vi "P4CMD Find All Providers.vi"(8 "error in (no error)":errorcluster) -> (0 "error out":errorcluster, 1 "additional data":string[](array[string]), 2 "provider locations":string[](array[string]), 3 "provider names":string[](array[string]))   [LabVIEW 2020, in "NI_SCC_P4CMD.lvlib"]
uses:
  <vilib>/SourceControl/Providers/P4CMD/NI_SCC_P4CMD.lvlib
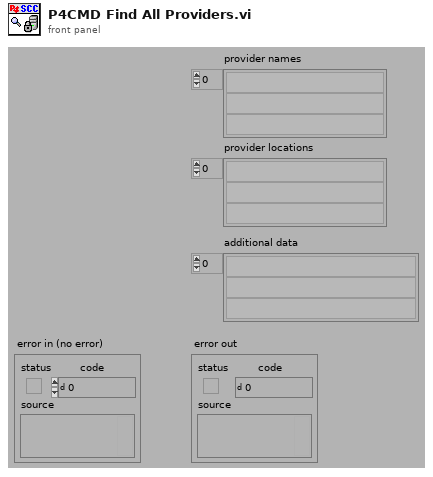
[diagram p1: front panel]
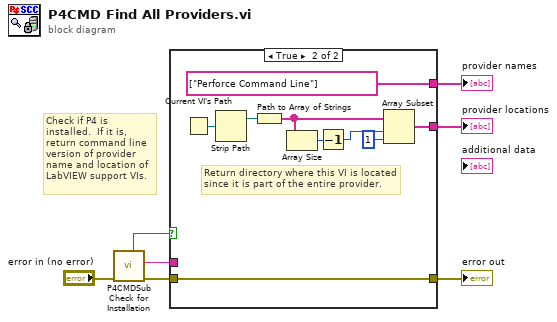
[diagram p0: block diagram]
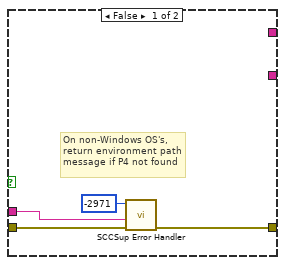
[diagram p2: hidden frame]
diagram:
  # "Check if P4 is installed.  If it is, return command line version of provider name and location of LabVIEW support VIs."
  n1 = call <vilib>:"P4CMDSub Check for Installation.vi"("error in (no error)"="error in (no error)") -> ("error out"=w2:errorcluster, "path info"=w4:string, "Perforce installed?"=w5:bool)  [unwired: 8 in]
  n2 = case shown="True" w5 {
    tunnel: [_ string[] ["Perforce Command Line"] ("provider names")] -> w7
    tunnel: w4 -> [w9 _]
    tunnel: [_ w12] -> w3
    tunnel: w2 -> [w11 w19]
    tunnel: [w10 w19] -> w1
    frame False {
      # "On non-Windows OS's, return environment path message if P4 not found"
      n3 = call <vilib>:"SCCSup Error Handler.vi"("error in (no error)"=w11, "additional message"=w9, "scc error code"=-2971 ("error code")) -> ("error out"=w10:errorcluster)  [unwired: 8 in]
    }
    frame True {
      # "Return directory where this VI is located since it is part of the entire provider."
      n4 = Current VI's Path() -> (path=w18:path)
      n5 = Strip Path(path=w18) -> (stripped path=w17:path)  [unwired: 1 out]
      n6 = Path to Array of Strings(0:w17) -> (2:w15:string[])  [unwired: 1 out]
      n7 = Array Size(array=w15) -> (size(s)=w16:i32)
      n8 = Decrement(x=w16) -> (x-1=w14:i32)
      n9 = Array Subset(array=w15, index=w14, length=1) -> (w12:string[])
    }
  }
  "error out" <- w1
  "provider names" <- w7
  "provider locations" <- w3
